vi "Get OFDM Impairments.vi"(8 "error in (no error)":errorcluster, 11 "niDTS WLAN INSTR TX in":refnum<class "niDTS WLAN INSTR TX.lvclass">) -> (0 "error out":errorcluster, 2 "OFDM Impairments":T1, 3 "niDTS WLAN INSTR TX out":refnum<class "niDTS WLAN INSTR TX.lvclass">)   [LabVIEW 2015, in "niDTS WLAN.lvlib" / "niDTS WLAN INSTR TX.lvclass"]
uses:
  niDTS WLAN INSTR TX.lvclass
  niDTS WLAN INSTR TX INC OFDM Impairments Results.ctl
  niDTS WLAN INSTR TX.lvclass/niDTS WLAN INSTR TX.ctl
  RiviInstDriver/niRfsaWlan/Objects/niRfsaWlan.lvclass
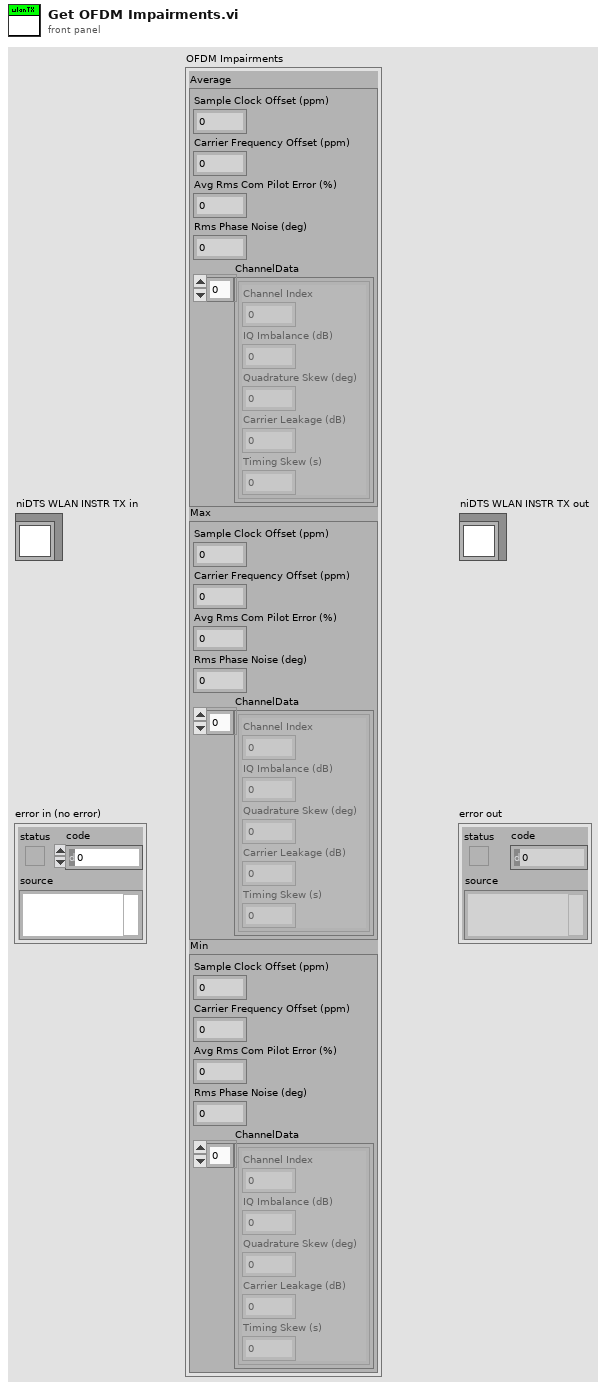
[diagram p1: front panel]
types:
  T1 = typedef "niDTS WLAN.lvlib/niDTS WLAN INSTR TX.lvclass/niDTS WLAN INSTR TX INC OFDM Impairments Results.ctl" = cluster{"Average":cluster{"Sample Clock Offset (ppm)":dbl, "Carrier Frequency Offset (ppm)":dbl, "Avg Rms Com Pilot Error (%)":dbl, "Rms Phase Noise (deg)":dbl, "ChannelData":cluster{"Channel Index":i32, "IQ Imbalance (dB)":dbl, "Quadrature Skew (deg)":dbl, "Carrier Leakage (dB)":dbl, "Timing Skew (s)":dbl}[]}, "Max":cluster{"Sample Clock Offset (ppm)":dbl, "Carrier Frequency Offset (ppm)":dbl, "Avg Rms Com Pilot Error (%)":dbl, "Rms Phase Noise (deg)":dbl, "ChannelData":cluster{"Channel Index":i32, "IQ Imbalance (dB)":dbl, "Quadrature Skew (deg)":dbl, "Carrier Leakage (dB)":dbl, "Timing Skew (s)":dbl}[]}, "Min":cluster{"Sample Clock Offset (ppm)":dbl, "Carrier Frequency Offset (ppm)":dbl, "Avg Rms Com Pilot Error (%)":dbl, "Rms Phase Noise (deg)":dbl, "ChannelData":cluster{"Channel Index":i32, "IQ Imbalance (dB)":dbl, "Quadrature Skew (deg)":dbl, "Carrier Leakage (dB)":dbl, "Timing Skew (s)":dbl}[]}}
  T2 = typedef "niRfsaWlan.lvclass/niRfsaWlan INC Handle.ctl" = refnum<data-value>
  T3 = typedef "niDTS WLAN.lvlib/niDTS WLAN Tx Test INC Parameters.ctl" = cluster{"Standard":T4, "DSSS Data Rate (Mbps)":T5, "OFDM Data Rate (Mbps)":T6, "MCS Index":i32, "N spatial streams":i32, "Chains":bool[], "BandWidth (Hz)":T7, "Channel":i32, "Gard Interval":T8, "FEC Coding":T9, "Dut Tx Power":dbl, "16 symbols":bool, "payload length bytes":i32, "idle interval":dbl, "External Attenuation":dbl[], "Acquisition Parameters ":T10, "TXP Measurement Parameters":T11, "ModAcc Measurement Paramaters":T12, "ModAcc DSSS Paramaters":T13, "SEM Measurement Parameters":T15, "OBW Measurement Parameters":T16, "DSSS Power Ramp":T17, "Enable Traces":bool}
  T4 = typedef "niDTS WLAN.lvlib/niDTS WLAN INC Standard.ctl" = enum16{"802.11 b DSSS", "802.11 a/g OFDM", "802.11 n HT", "802.11 ac VHT"}
  T5 = typedef "niDTS WLAN.lvlib/niDTS WLAN INC DSSS Data Rate.ctl" = enum16{"1", "2", "5.5", "11"}
  T6 = typedef "niDTS WLAN.lvlib/niDTS WLAN INC OFDM Data Rate.ctl" = enum16{"6", "9", "12", "18", "24", "36", "48", "54"}
  T7 = typedef "niDTS WLAN.lvlib/niDTS WLAN INC CH BW.ctl" = enum16{"20 MHz", "40 MHz", "80 MHz", "160 MHz"}
  T8 = typedef "niDTS WLAN.lvlib/niDTS WLAN INC GI.ctl" = enum16{"LONG", "SHORT"}
  T9 = typedef "niDTS WLAN.lvlib/niDTS WLAN INC FEC Coding.ctl" = enum16{"BCC", "LDPC"}
  T10 = typedef "niDTS WLAN.lvlib/niDTS WLAN DUT INC Acquisition Parameters.ctl" = cluster{"Acquisition Length Mode":enum16{"AUTO", "MANUAL"}, "Acquisition Length (s)":dbl, "Auto Level":bool}
  T11 = typedef "niDTS WLAN.lvlib/niDTS WLAN INC TXP Measurement Parameters.ctl" = cluster{"TXP Power Enable":bool, "TXP Averages":i32}
  T12 = typedef "niDTS WLAN.lvlib/niDTS WLAN INC ModAcc Measurement Parameters.ctl" = cluster{"ModAcc Enable":bool, "Header Detection":enum16{"MANUAL", "FIRST", "ALL"}, "Averages":i32, "Amplitude Tracking":bool, "Channel Tracking":bool, "Time Tracking":bool, "Phase Tracking":enum16{"NONE", "STANDARD", "CSF", "INSTANT"}, "Clock Offset Est":bool, "Impairments Est":bool, "CFO Estimation":enum16{"PAMBLE", "PDATA"}}
  T13 = typedef "niDTS WLAN.lvlib/niDTS WLAN INC DSSS ModAcc Measurement Parameters.ctl" = cluster{"DC Offset Compensation":bool, "Equalization":bool, "Phase Tracking":bool, "Chip Start Location":i16, "Max Chips Used":i16, "Pulse Shaping FilterType":T14, "Pulse Shaping Filter Coefficient":dbl}
  T14 = typedef "niDTS WLAN.lvlib/niDTS WLAN INC Pulse Shaping Filter Type.ctl" = enum16{"NONE", "RCOSINE", "RRCOSINE", "GAUSSIAN"}
  T15 = typedef "niDTS WLAN.lvlib/niDTS WLAN INC SEM Measurement Parameters.ctl" = cluster{"SEM Enable":bool, "SEM Averages":i32, "Auto Span Enable":bool, "Frequency Span (Hz)":dbl, "Measurement Type":enum16{"Standard", "Legacy", "Custom"}, "Mask Frequencies (Hz)":dbl[], "Mask Power Offsets (dB)":dbl[]}
  T16 = typedef "niDTS WLAN.lvlib/niDTS WLAN INC OBW Measurement Parameters.ctl" = cluster{"OBW Enable":bool, "OBW Averages":i32}
  T17 = typedef "niDTS WLAN.lvlib/niDTS WLAN INC DSSS Power Ramp Parameters.ctl" = cluster{"Power Ramp Enable":bool, "Averages":i32, "Thresholds":cluster{"Up Low (%)":dbl, "Down Low (%)":dbl, "Up High (%)":dbl, "Down High (%)":dbl}}
  T18 = cluster{"SampleClockOffset":dbl, "CarrierFrequencyOffset":dbl, "AvgRmsComPilotErr":dbl, "RmsPhaseNoise":dbl, "ChannelData":cluster{"ChannelIndex":i32, "ChannelIqImbalance":dbl, "ChannelQuadratureSkew":dbl, "ChannelCarrierFreqLeakage":dbl, "ChannelTimingSkew":dbl}[]}
  T19 = cluster{"AvgImpairmentResults":cluster{"SampleClockOffset":dbl, "CarrierFrequencyOffset":dbl, "AvgRmsComPilotErr":dbl, "RmsPhaseNoise":dbl, "ChannelData":cluster{"ChannelIndex":i32, "ChannelIqImbalance":dbl, "ChannelQuadratureSkew":dbl, "ChannelCarrierFreqLeakage":dbl, "ChannelTimingSkew":dbl}[]}, "MaxImpairmentResults":cluster{"SampleClockOffset":dbl, "CarrierFrequencyOffset":dbl, "AvgRmsComPilotErr":dbl, "RmsPhaseNoise":dbl, "ChannelData":cluster{"ChannelIndex":i32, "ChannelIqImbalance":dbl, "ChannelQuadratureSkew":dbl, "ChannelCarrierFreqLeakage":dbl, "ChannelTimingSkew":dbl}[]}, "MinImpairmentResults":cluster{"SampleClockOffset":dbl, "CarrierFrequencyOffset":dbl, "AvgRmsComPilotErr":dbl, "RmsPhaseNoise":dbl, "ChannelData":cluster{"ChannelIndex":i32, "ChannelIqImbalance":dbl, "ChannelQuadratureSkew":dbl, "ChannelCarrierFreqLeakage":dbl, "ChannelTimingSkew":dbl}[]}}
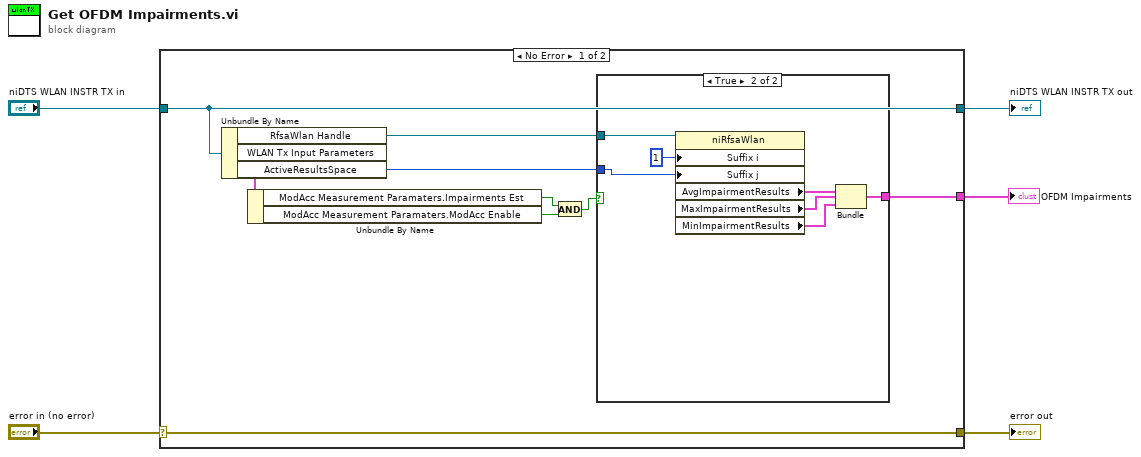
[diagram p0: block diagram]
diagram:
  n1 = case shown="No Error" "error in (no error)" {
    selector: "error in (no error)" -> [w14 w23]
    tunnel: [w14 w23] -> w4
    tunnel: [w13 w22] -> w2
    tunnel: "niDTS WLAN INSTR TX in" -> [w13 w22]
    tunnel: [w10 _] -> w1
    frame No Error {
      n2 = Unbundle By Name(w13) -> ("RfsaWlan Handle"=w11:T2, "WLAN Tx Input Parameters"=w12:T3, "ActiveResultsSpace"=w9:u8)
      n3 = Unbundle By Name(w12) -> ("ModAcc Measurement Paramaters.Impairments Est"=w6:bool, "ModAcc Measurement Paramaters.ModAcc Enable"=w7:bool)
      n4 = And(x=w6, y=w7) -> (x .and. y?=w8:bool)
      n5 = case shown="True" w8 {
        tunnel: w11 -> [_ w21]
        tunnel: [_ w16] -> w10
        tunnel: w9 -> [_ w15]
        frame False {
        }
        frame True {
          n6 = property class="niRfsaWlan"(reference=w21, "Suffix i"=1 ("Active Channel:Suffix i"), "Suffix j"=w15) -> ("AvgImpairmentResults"=w19:T18, "MaxImpairmentResults"=w18:T18, "MinImpairmentResults"=w17:T18)  [unwired: 1 in, 2 out]
          n7 = Bundle("AvgImpairmentResults"=w19, "MaxImpairmentResults"=w18, "MinImpairmentResults"=w17) -> (w16:T19)  [unwired: 1 in]
        }
      }
    }
    frame Error {
    }
  }
  "error out" <- w4
  "niDTS WLAN INSTR TX out" <- w2
  "OFDM Impairments" <- w1
